vi "GetDataFromFile.vi"(0 "FileName":string, 5 "error in (no error)":errorcluster) -> (14 "FileData":T1, 16 "file or folder exists?":bool, 19 "error out":errorcluster)   [LabVIEW 2014, in "IndoorData.lvclass"]
uses:
  IndoorData.lvclass
  BufferedReadings.ctl
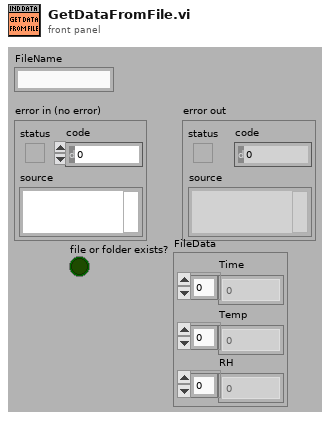
[diagram p1: front panel]
types:
  T1 = typedef "IndoorData.lvclass/BufferedReadings.ctl" = cluster{"Time":dbl[], "Temp":dbl[], "RH":dbl[]}
  T2 = typedef "IndoorData.lvclass/ObjectAttributes.ctl" = cluster{"DebugData":T3, "Actual":T4, "BufferedReadings":T1, "AVGReadings":T1, "LogFolder":path, "FirstLog?":bool, "MinMaxFile":path}
  T3 = typedef "IndoorData.lvclass/DebugData.ctl" = cluster{"Rev":string, "Location":string, "LoopIdx":i32, "PiCoreTemp":dbl, "Error":errorcluster}
  T4 = typedef "IndoorData.lvclass/ActualValues.ctl" = cluster{"Time":dbl, "Temp":dbl, "RH":dbl}
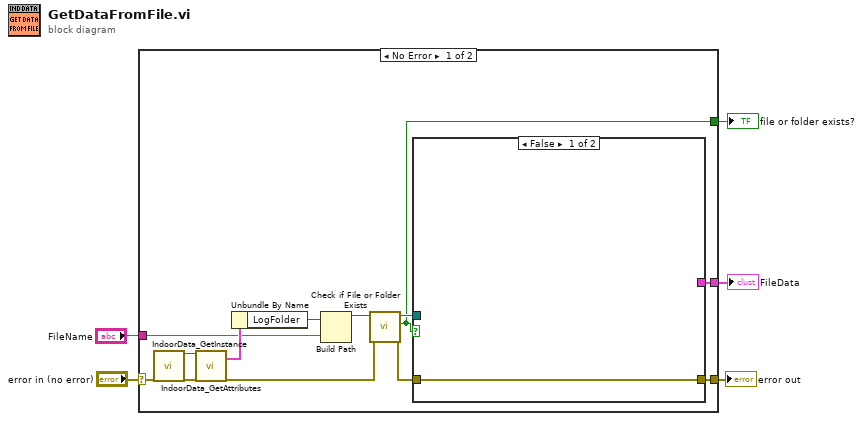
[diagram p0: block diagram]
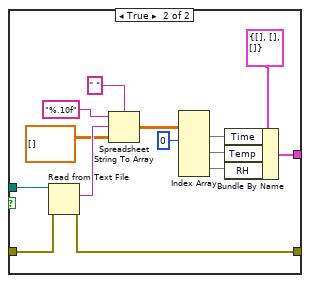
[diagram p2: hidden frame]
diagram:
  n1 = case shown="No Error" "error in (no error)" {
    selector: "error in (no error)" -> [w16 w34]
    tunnel: [w12 w34] -> w4
    tunnel: "FileName" -> [w13 _]
    tunnel: [w11 _] -> w2
    tunnel: [w6 _] -> w1
    frame No Error {
      n2 = call "IndoorData_GetInstance.vi"("error in (no error)"=w16) -> ("reference out"=w18:refnum<class "IndoorData.lvclass">, "error out"=w15:errorcluster)  [unwired: 14 in, 3 out]
      n3 = call "IndoorData_GetAttributes.vi"("reference in"=w18, "error in (no error)"=w15) -> ("Data"=w17:T2, "error out"=w8:errorcluster)  [unwired: 14 in, 2 out]
      n4 = Unbundle By Name(w17) -> ("LogFolder"=w14:path)
      n5 = Build Path(base path=w14, name or relative path=w13) -> (appended path=w10:path)
      n6 = call <vilib>:"Check if File or Folder Exists.vi"("error in (no error)"=w8, "path"=w10) -> ("error out"=w7:errorcluster, "file or folder exists?"=w6:bool, "dup path"=w9:path)  [unwired: 7 in]
      n7 = case shown="False" w6 {
        tunnel: [w19 w24] -> w12
        tunnel: [_ w22] -> w11
        tunnel: w9 -> [_ w21]
        tunnel: w7 -> [w19 w20]
        frame False {
        }
        frame True {
          n8 = Read from Text File(file (use dialog)=w21, error in=w20) -> (text=w33:string, error out=w24:errorcluster)  [unwired: 2 in, 2 out]
          n9 = Spreadsheet String To Array(delimiter (Tab)=" ", format string="%.10f", spreadsheet string=w33, array type (2D Dbl)=dbl[][] []) -> (array=w29:dbl[][])
          n10 = Index Array(array=w29, index (col) #1=0 ("disabled index (col)")) -> (element #1=w27:dbl[], element #2=w26:dbl[], element #3=w25:dbl[])  [unwired: 5 in]
          n11 = Bundle By Name(cluster=T1 {"Time"=[], "Temp"=[], "RH"=[]} ("BufferedReadings"), "Time"=w27, "Temp"=w26, "RH"=w25) -> (w22:T1)
        }
      }
    }
    frame Error {
    }
  }
  "error out" <- w4
  "FileData" <- w2
  "file or folder exists?" <- w1
